vi "移动完成.vi"(0 "原始X":u8, 1 "移动后的X":u8, 2 "输入的棋盘":T1, 3 "原始Y":u8, 4 "移动后的Y":u8) -> (5 "输出的棋盘":T1, 6 "结果":string)   [LabVIEW 2017]
panel:
  out "输出数组":bool[][](array[boolean])
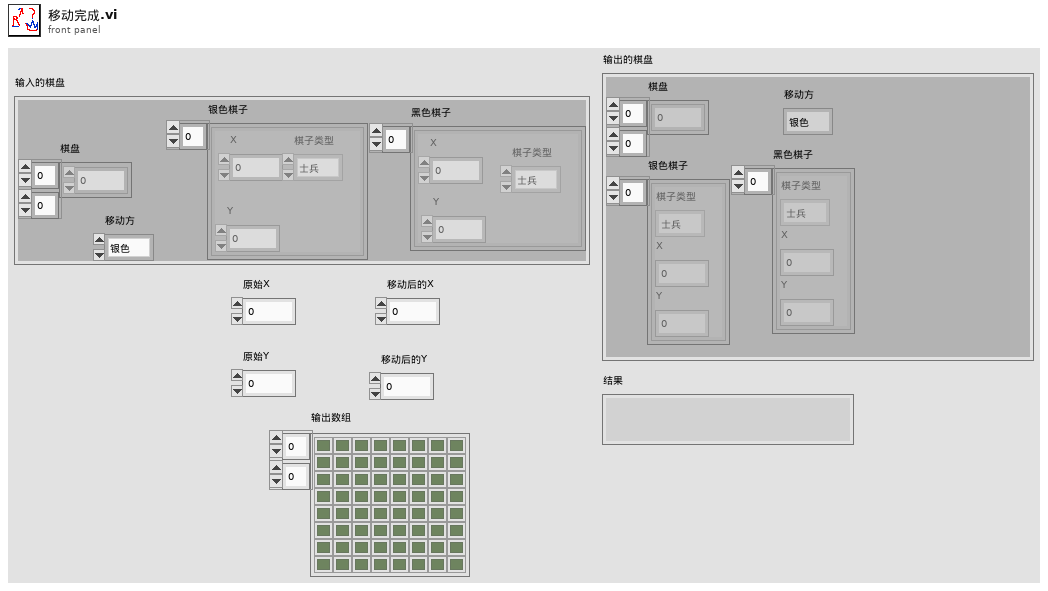
[diagram p1: front panel]
types:
  T1 = cluster{"棋盘":u16[][], "银色棋子":cluster{"棋子类型":enum16{"士兵", "骑士", "主教", "战车", "皇后", "国王", "空"}, "X":u8, "Y":u8}[], "黑色棋子":cluster{"棋子类型":enum16{"士兵", "骑士", "主教", "战车", "皇后", "国王", "空"}, "X":u8, "Y":u8}[], "移动方":enum16{"银色", "黑色"}}
  T2 = cluster{"棋子类型":enum16{"士兵", "骑士", "主教", "战车", "皇后", "国王", "空"}, "X":u8, "Y":u8}
  T3 = cluster{"棋子类型":enum16{"士兵", "骑士", "主教", "战车", "皇后", "国王", "空"}, "X":u8, "Y":u8}[]
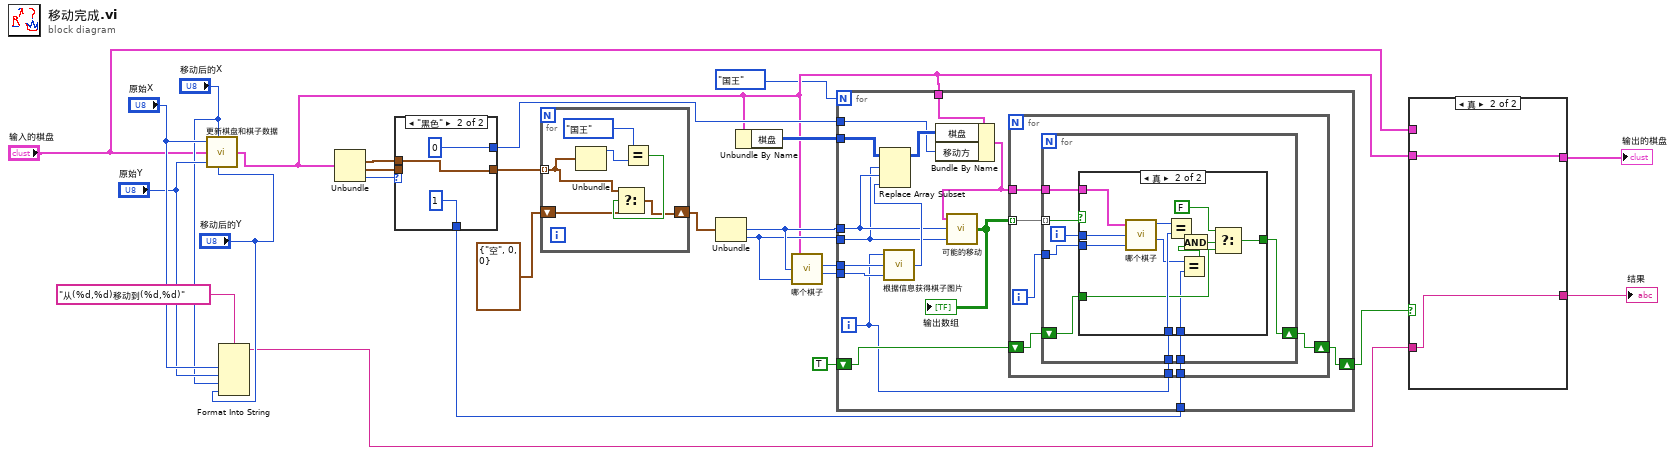
[diagram p0: block diagram]
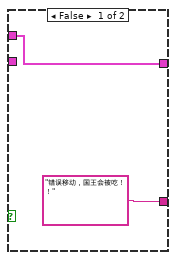
[diagram p2: hidden frame]
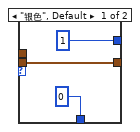
[diagram p4: hidden frame]
diagram:
  n1 = call "更新棋盘和棋子数据.vi"("原始位置X"="原始X", "到达的X"="移动后的X", "游戏"="输入的棋盘", "原始位置Y"="原始Y", "到达的Y"="移动后的Y") -> ("游戏 2"=w8:T1)
  n2 = Format Into String(format string="从(%d,%d)移动到(%d,%d)" ("初始字符串"), "原始X", "原始Y", "移动后的X", "移动后的Y") -> (resulting string=w7:string)  [unwired: 2 in, 1 out]
  n3 = Unbundle(w8) -> ("银色棋子"=w20:T3, "黑色棋子"=w21:T3, "移动方"=w22:enum16{"银色", "黑色"})  [unwired: 1 out]
  n4 = case shown="\"黑色\"" w22 {
    tunnel: w21 -> [w29 _]
    tunnel: [w29 w32] -> w19
    tunnel: w20 -> [_ w32]
    tunnel: [1 0] -> w12
    tunnel: [0 1] -> w10
    frame "银色", Default {
    }
    frame "黑色" {
    }
  }
  n5 = for {
    tunnel: w19 -> [w38] mode=indexing
    shift-right: [w34] -> w18
    shift-left: T2 {"棋子类型"=enum."空", "X"=0, "Y"=0} -> [w35]
    n6 = Unbundle(w38) -> ("棋子类型"=w36:enum16{"士兵", "骑士", "主教", "战车", "皇后", "国王", "空"})  [unwired: 2 out]
    n7 = Equal?(x=enum16{"士兵", "骑士", "主教", "战车", "皇后", "国王", "空"}."国王", y=w36) -> (x = y?=w37:bool)
    n8 = Select(t=w38, s=w37, f=w35) -> (s? t:f=w34:T2)
  }
  n9 = Unbundle(w18) -> ("X"=w17:u8, "Y"=w16:u8)  [unwired: 1 out]
  n10 = Unbundle By Name(w8) -> ("棋盘"=w13:u16[][])
  n11 = call "哪个棋子.vi"("游戏"=w8, "X"=w17, "Y"=w16) -> ("背景颜色"=w15:enum16{"白色", "绿色"}, "棋子颜色"=w14:enum16{"银色", "黑色"})  [unwired: 2 out]
  n12 = for {
    N: enum16{"士兵", "骑士", "主教", "战车", "皇后", "国王", "空"}."国王" ("x") -> [_]
    tunnel: w17 -> [w45]
    tunnel: w16 -> [w44]
    tunnel: w15 -> [w52]
    tunnel: w14 -> [w51]
    tunnel: w8 -> [w48]
    tunnel: w13 -> [w53]
    tunnel: w12 -> [w47]
    shift-right: [w40] -> w9
    shift-left: TRUE -> [w43]
    tunnel: w10 -> [w39]
    i -> [w41]
    n13 = call "根据信息获得棋子图片.vi"("棋子颜色"=w51, "背景颜色"=w52, "棋子类型"=w41) -> ("棋子"=w50:u16)
    n14 = Replace Array Subset(array=w53, new element=w50, index (row)=w44, index (col)=w45) -> (w49:u16[][])
    n15 = Bundle By Name(cluster=w48, "棋盘"=w49, "移动方"=w47) -> (w42:T1)
    n16 = call "可能的移动.vi"("Y"=w44, "X"=w45, "游戏"=w42) -> ("输出数组"=w46:bool[][])
    "输出数组" <- w46
    n17 = for {
      tunnel: w46 -> [w60] mode=indexing
      shift-right: [w55] -> w40
      shift-left: w43 -> [w56]
      tunnel: w42 -> [w58]
      tunnel: w41 -> [w57]
      tunnel: w39 -> [w54]
      i -> [w59]
      n18 = for {
        tunnel: w60 -> [w67] mode=indexing
        tunnel: w59 -> [w66]
        tunnel: w58 -> [w68]
        tunnel: w57 -> [w64]
        shift-right: [w62] -> w55
        shift-left: w56 -> [w63]
        tunnel: w54 -> [w61]
        i -> [w65]
        n19 = case shown="真" w67 {
          tunnel: w68 -> [_ w82]
          tunnel: w66 -> [_ w81]
          tunnel: w65 -> [_ w80]
          tunnel: w64 -> [_ w78]
          tunnel: w63 -> [w69 w75]
          tunnel: [w69 w76] -> w62
          tunnel: w61 -> [_ w73]
          frame False {
          }
          frame True {
            n20 = call "哪个棋子.vi"("游戏"=w82, "X"=w80, "Y"=w81) -> ("棋子类型"=w79:enum16{"士兵", "骑士", "主教", "战车", "皇后", "国王", "空"}, "棋子颜色"=w74:enum16{"银色", "黑色"})  [unwired: 2 out]
            n21 = Equal?(x=w79, y=w78) -> (x = y?=w71:bool)
            n22 = Equal?(x=w74, y=w73) -> (x = y?=w70:bool)
            n23 = And(x=w71, y=w70) -> (x .and. y?=w72:bool)
            n24 = Select(t=FALSE, s=w72, f=w75) -> (s? t:f=w76:bool)
          }
        }
      }
    }
  }
  n25 = case shown="真" w9 {
    tunnel: "输入的棋盘" -> [w84 _]
    tunnel: w8 -> [_ w86]
    tunnel: w7 -> [_ w85]
    tunnel: [w84 w86] -> w2
    tunnel: ["错误移动，国王会被吃！！" w85] -> w1
    frame False {
    }
    frame True {
    }
  }
  "输出的棋盘" <- w2
  "结果" <- w1
